vi "get reserving node.vi"(8 "error in (no error)":errorcluster, 10 "FPGA Resource":T2, 11 "Item Ref in":T1 format="%.0x") -> (0 "error out":errorcluster, 1 "Dependent Node Ref":T1=18446744073709551615 format="%.0x", 3 "Item Ref out":T1 format="%.0x", 4 "Found":bool)   [LabVIEW 2016, in "FPGA RM System Definition API.lvlib"]
uses:
  System Definition/FPGA RM System Definition API.lvlib
  fpga resource.ctl
  Channel Type.ctl
  <vilib>/NI Veristand/Custom Device API/Custom Device Item Ref.ctl
  <vilib>/NI VeriStand/Custom Device API/Custom Device API.lvlib
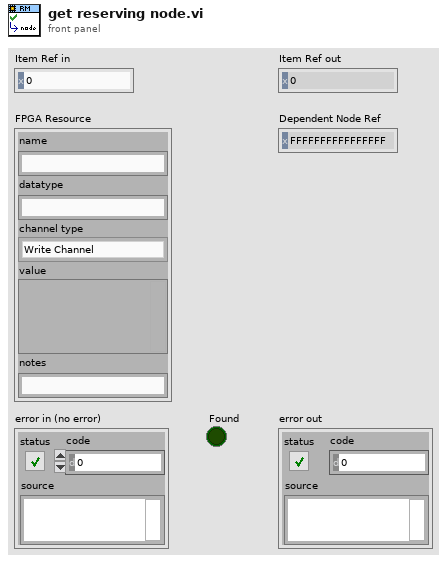
[diagram p1: front panel]
types:
  T1 = typedef "Custom Device API.lvlib/Custom Device Item Ref.ctl" = u64
  T2 = typedef "FPGA RM System Definition API.lvlib/fpga resource.ctl" = cluster{"name":string, "datatype":string, "channel type":T3, "value":variant, "notes":string}
  T3 = typedef "FPGA RM System Definition API.lvlib/Channel Type.ctl" = enum16{"Write Channel", "Read Channel", "Write Waveform", "Read Waveform"}
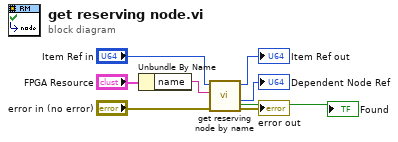
[diagram p0: block diagram]
diagram:
  n1 = Unbundle By Name("FPGA Resource") -> ("name"=w6:string)
  n2 = call "get reserving node by name.vi"("error in (no error)"="error in (no error)", "name"=w6, "Item Ref in"="Item Ref in") -> ("error out"=→"error out":errorcluster, "Dependent Node Ref"=→"Dependent Node Ref":T1, "Item Ref out"=→"Item Ref out":T1, "Found"=→"Found":bool)  [unwired: 5 in]
